vi "Z900_navX_Get_SystemInformation_Status.vi"(8 "error in (no error)":errorcluster, 11 "navX Device":T4={"Interface"={"Protocol"=enum."SERIAL", "Update Rate (4Hz-100Hz)"=4, "navX Open TypeDef"=variant}, "Notify Packet"=refnum, "Loop VI Refnum"=refnum, "Ready to Close Occurrence Refnum"=refnum} {"Interface"."Update Rate (4Hz-100Hz)" min=4 max=60 step=1}) -> (0 "error out":errorcluster, 1 "Connected":bool, 2 "Status":T3 {"OP Status" items=["INITIALIZING", "SELFTEST_IN_PROGRESS", "ERROR", "IMU_AUTOCAL_IN_PROGRESS", "NORMAL"]; "Calibration Status" items=["IMU_CAL_STATE_MASK"=3, "IMU_CAL_STATE_INPROGRESS"=0, "IMU_CAL_STATE_ACCUMULATE"=1, "IMU_CAL_STATE_COMPLETE"=2]}, 3 "navX Device":T4={"Interface"={"Protocol"=enum."SERIAL", "Update Rate (4Hz-100Hz)"=4, "navX Open TypeDef"=variant}, "Notify Packet"=refnum, "Loop VI Refnum"=refnum, "Ready to Close Occurrence Refnum"=refnum} {"Interface"."Update Rate (4Hz-100Hz)" min=4 max=60 step=1})   [LabVIEW 2015, in "Apple Pi Gyro Library.lvlib" / "navX Library v2.lvlib"]
doc: "This navX VI returns the current status of the navX."
uses:
  navX Library v2.lvlib
  TypeDefs/Z900_navX_DeviceTypeDef.ctl
  TypeDefs/Z900_navX_ProtocolTypeDef.ctl
  TypeDefs/Z900_navX_NotifyPacketTypeDef.ctl
  TypeDefs/Z900_navX_ActionTypeDef.ctl
  TypeDefs/Flags/Z900_navX_Flags_OpStatusTypeDef.ctl
  TypeDefs/Flags/Z900_navX_Flags_CalibrationStatusTypeDef.ctl
  TypeDefs/Z900_navX_DeviceRegisters.ctl
  TypeDefs/Flags/Z900_navX_Flags_SelfTestStatusTypeDef.ctl
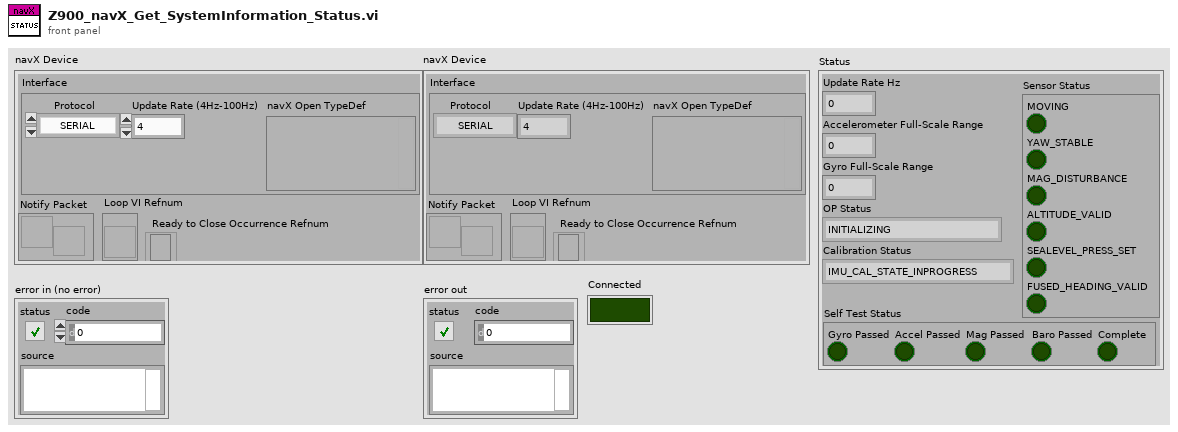
[diagram p1: front panel]
types:
  T1 = typedef "Apple Pi Gyro Library.lvlib/navX Library v2.lvlib/Z900_navX_Flags_OpStatusTypeDef.ctl" = u8
  T2 = typedef "Apple Pi Gyro Library.lvlib/navX Library v2.lvlib/Z900_navX_Flags_CalibrationStatusTypeDef.ctl" = u8
  T3 = cluster{"Update Rate Hz":u8, "Accelerometer Full-Scale Range":u8, "Gyro Full-Scale Range":u16, "OP Status":T1, "Calibration Status":T2, "Sensor Status":cluster{"MOVING":bool, "YAW_STABLE":bool, "MAG_DISTURBANCE":bool, "ALTITUDE_VALID":bool, "SEALEVEL_PRESS_SET":bool, "FUSED_HEADING_VALID":bool}, "Self Test Status":cluster{"Gyro Passed":bool, "Accel Passed":bool, "Mag Passed":bool, "Baro Passed":bool, "Complete":bool}}
  T4 = typedef "Apple Pi Gyro Library.lvlib/navX Library v2.lvlib/Z900_navX_DeviceTypeDef.ctl" = cluster{"Interface":cluster{"Protocol":T5, "Update Rate (4Hz-100Hz)":u8, "navX Open TypeDef":variant}, "Notify Packet":refnum<notifier>, "Loop VI Refnum":refnum<vi>, "Ready to Close Occurrence Refnum":refnum<k4>}
  T5 = typedef "Apple Pi Gyro Library.lvlib/navX Library v2.lvlib/Z900_navX_ProtocolTypeDef.ctl" = enum16{"SERIAL", "I2C", "SPI"}
  T6 = cluster{"MOVING":bool, "YAW_STABLE":bool, "MAG_DISTURBANCE":bool, "ALTITUDE_VALID":bool, "SEALEVEL_PRESS_SET":bool, "FUSED_HEADING_VALID":bool}
  T7 = typedef "Apple Pi Gyro Library.lvlib/navX Library v2.lvlib/Z900_navX_DeviceRegisters.ctl" = u8
  T8 = cluster{"Gyro Passed":bool, "Accel Passed":bool, "Mag Passed":bool, "Baro Passed":bool, "Complete":bool}
  T9 = typedef "Apple Pi Gyro Library.lvlib/navX Library v2.lvlib/Z900_navX_Flags_SelfTestStatusTypeDef.ctl" = u8
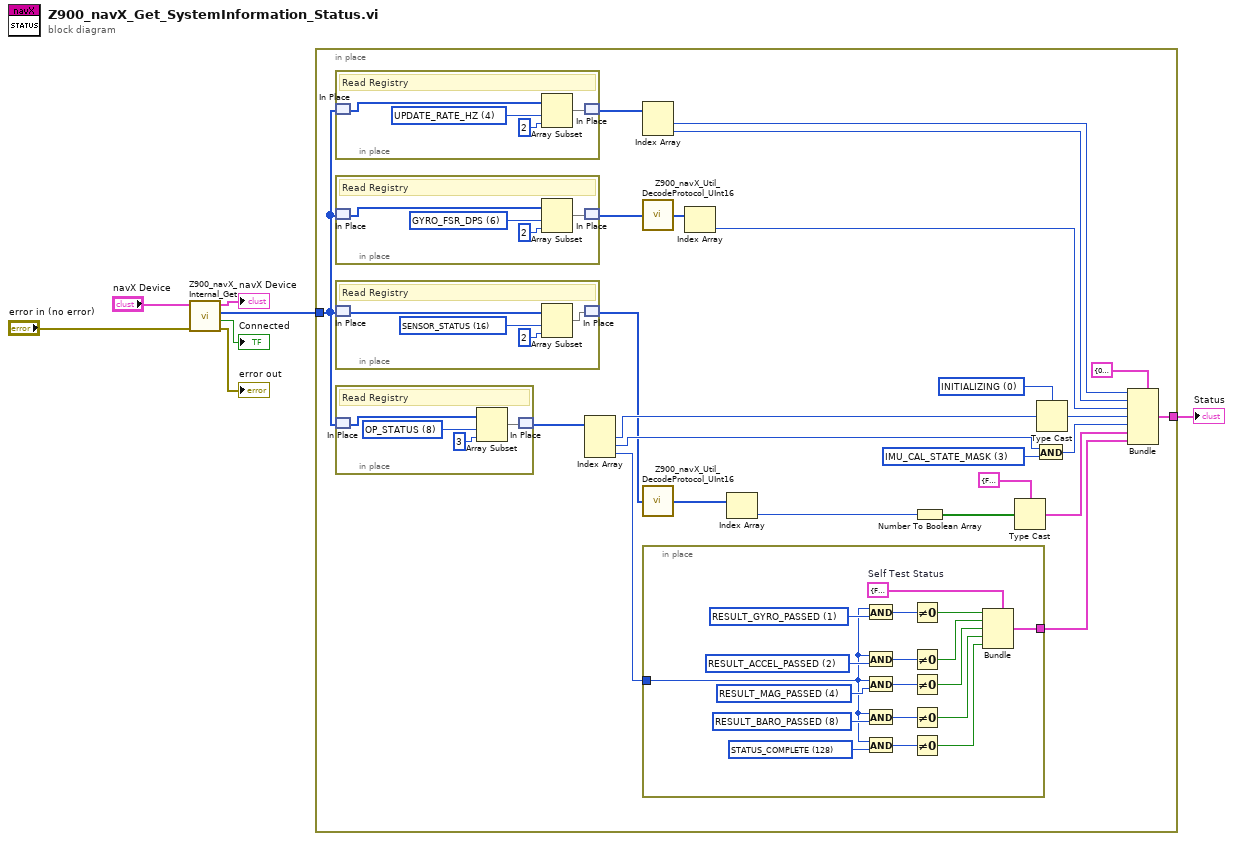
[diagram p0: block diagram]
diagram:
  n1 = call "Z900_navX_Internal_Get.vi"("error in (no error)"="error in (no error)", "navX Device"="navX Device") -> ("error out"=→"error out":errorcluster, "Connected"=→"Connected":bool, "Registry"=w3:u8[], "navX Device"=→"navX Device":T4)  [unwired: 6 in]
  n2 = in-place {
    in-place-border: w3 -> [w16]
    in-place-border: [w23] -> w1
    w27 = T2 3 items=["IMU_CAL_STATE_MASK"=3, "IMU_CAL_STATE_INPROGRESS"=0, "IMU_CAL_STATE_ACCUMULATE"=1, "IMU_CAL_STATE_COMPLETE"=2] ("CalibrationStatus")
    w29 = T1 0 items=["INITIALIZING", "SELFTEST_IN_PROGRESS", "ERROR", "IMU_AUTOCAL_IN_PROGRESS", "NORMAL"] ("OP Status")
    n3 = in-place {
      w52 = T7 4 items=["WHOAMI"=0, "HW_REV"=1, "FW_VER_MAJOR"=2, "FW_VER_MINOR"=3, "UPDATE_RATE_HZ"=4, "ACCEL_FSR_G"=5, "GYRO_FSR_DPS"=6, "OP_STATUS"=8, "CAL_STATUS"=9, "SELFTEST_STATUS"=10, "CAPABILITY_FLAGS_L"=11, "CAPABILITY_FLAGS_H"=12, "SENSOR_STATUS"=16, "TIMESTAMP"=18, "YAW"=22, "ROLL"=24, "PITCH"=26, "HEADING"=28, "FUSED_HEADING"=30, "ALTITUDE_I"=32, "ALTITUDE_D"=34, "LINERA_ACC_X"=36, "LINERA_ACC_Y"=38, "LINERA_ACC_Z"=40, "QUAT_W"=42, "QUAT_X"=44, "QUAT_Y"=46, "QUAT_Z"=48, "MPU_TEMP_C"=50, "GYRO_X"=52, "GYRO_Y"=54, "GYRO_Z"=56, "ACC_X"=58, "ACC_Y"=60, "ACC_Z"=62, "MAG_X"=64, "MAG_Y"=66, "MAG_Z"=68, "PRESSURE_I"=70, "PRESSURE_D"=72, "PRESSURE_TEMP"=74, "YAW_OFFSET"=76, "QUAT_OFFSET_W"=78, "QUAT_OFFSET_X"=80, "QUAT_OFFSET_Y"=82, "QUAT_OFFSET_Z"=84, "INTEGRATION_CONTROL"=86, "VELOCITY_X"=88, "VELOCITY_Y"=92, "VELOCITY_Z"=96, "DISPLACMENT_X"=100, "DISPLACMENT_Y"=104, "DISPLACEMENT_Z"=108] ("Device Register")
      # "Read Registry"
      n4 = in-place-match #1(w16) -> (w50:u8[])
      n5 = Array Subset(array=w50, index=w52, length=2) -> (w51:u8[])
      n6 = in-place-match #1(w51) -> (w15:u8[])
    }
    n7 = in-place {
      w64 = T7 6 items=["WHOAMI"=0, "HW_REV"=1, "FW_VER_MAJOR"=2, "FW_VER_MINOR"=3, "UPDATE_RATE_HZ"=4, "ACCEL_FSR_G"=5, "GYRO_FSR_DPS"=6, "OP_STATUS"=8, "CAL_STATUS"=9, "SELFTEST_STATUS"=10, "CAPABILITY_FLAGS_L"=11, "CAPABILITY_FLAGS_H"=12, "SENSOR_STATUS"=16, "TIMESTAMP"=18, "YAW"=22, "ROLL"=24, "PITCH"=26, "HEADING"=28, "FUSED_HEADING"=30, "ALTITUDE_I"=32, "ALTITUDE_D"=34, "LINERA_ACC_X"=36, "LINERA_ACC_Y"=38, "LINERA_ACC_Z"=40, "QUAT_W"=42, "QUAT_X"=44, "QUAT_Y"=46, "QUAT_Z"=48, "MPU_TEMP_C"=50, "GYRO_X"=52, "GYRO_Y"=54, "GYRO_Z"=56, "ACC_X"=58, "ACC_Y"=60, "ACC_Z"=62, "MAG_X"=64, "MAG_Y"=66, "MAG_Z"=68, "PRESSURE_I"=70, "PRESSURE_D"=72, "PRESSURE_TEMP"=74, "YAW_OFFSET"=76, "QUAT_OFFSET_W"=78, "QUAT_OFFSET_X"=80, "QUAT_OFFSET_Y"=82, "QUAT_OFFSET_Z"=84, "INTEGRATION_CONTROL"=86, "VELOCITY_X"=88, "VELOCITY_Y"=92, "VELOCITY_Z"=96, "DISPLACMENT_X"=100, "DISPLACMENT_Y"=104, "DISPLACEMENT_Z"=108] ("Device Register")
      # "Read Registry"
      n8 = in-place-match #2(w16) -> (w62:u8[])
      n9 = Array Subset(array=w62, index=w64, length=2) -> (w63:u8[])
      n10 = in-place-match #2(w63) -> (w17:u8[])
    }
    n11 = in-place {
      w56 = T7 16 items=["WHOAMI"=0, "HW_REV"=1, "FW_VER_MAJOR"=2, "FW_VER_MINOR"=3, "UPDATE_RATE_HZ"=4, "ACCEL_FSR_G"=5, "GYRO_FSR_DPS"=6, "OP_STATUS"=8, "CAL_STATUS"=9, "SELFTEST_STATUS"=10, "CAPABILITY_FLAGS_L"=11, "CAPABILITY_FLAGS_H"=12, "SENSOR_STATUS"=16, "TIMESTAMP"=18, "YAW"=22, "ROLL"=24, "PITCH"=26, "HEADING"=28, "FUSED_HEADING"=30, "ALTITUDE_I"=32, "ALTITUDE_D"=34, "LINERA_ACC_X"=36, "LINERA_ACC_Y"=38, "LINERA_ACC_Z"=40, "QUAT_W"=42, "QUAT_X"=44, "QUAT_Y"=46, "QUAT_Z"=48, "MPU_TEMP_C"=50, "GYRO_X"=52, "GYRO_Y"=54, "GYRO_Z"=56, "ACC_X"=58, "ACC_Y"=60, "ACC_Z"=62, "MAG_X"=64, "MAG_Y"=66, "MAG_Z"=68, "PRESSURE_I"=70, "PRESSURE_D"=72, "PRESSURE_TEMP"=74, "YAW_OFFSET"=76, "QUAT_OFFSET_W"=78, "QUAT_OFFSET_X"=80, "QUAT_OFFSET_Y"=82, "QUAT_OFFSET_Z"=84, "INTEGRATION_CONTROL"=86, "VELOCITY_X"=88, "VELOCITY_Y"=92, "VELOCITY_Z"=96, "DISPLACMENT_X"=100, "DISPLACMENT_Y"=104, "DISPLACEMENT_Z"=108] ("Device Register")
      # "Read Registry"
      n12 = in-place-match #3(w16) -> (w54:u8[])
      n13 = Array Subset(array=w54, index=w56, length=2) -> (w55:u8[])
      n14 = in-place-match #3(w55) -> (w22:u8[])
    }
    n15 = in-place {
      w60 = T7 8 items=["WHOAMI"=0, "HW_REV"=1, "FW_VER_MAJOR"=2, "FW_VER_MINOR"=3, "UPDATE_RATE_HZ"=4, "ACCEL_FSR_G"=5, "GYRO_FSR_DPS"=6, "OP_STATUS"=8, "CAL_STATUS"=9, "SELFTEST_STATUS"=10, "CAPABILITY_FLAGS_L"=11, "CAPABILITY_FLAGS_H"=12, "SENSOR_STATUS"=16, "TIMESTAMP"=18, "YAW"=22, "ROLL"=24, "PITCH"=26, "HEADING"=28, "FUSED_HEADING"=30, "ALTITUDE_I"=32, "ALTITUDE_D"=34, "LINERA_ACC_X"=36, "LINERA_ACC_Y"=38, "LINERA_ACC_Z"=40, "QUAT_W"=42, "QUAT_X"=44, "QUAT_Y"=46, "QUAT_Z"=48, "MPU_TEMP_C"=50, "GYRO_X"=52, "GYRO_Y"=54, "GYRO_Z"=56, "ACC_X"=58, "ACC_Y"=60, "ACC_Z"=62, "MAG_X"=64, "MAG_Y"=66, "MAG_Z"=68, "PRESSURE_I"=70, "PRESSURE_D"=72, "PRESSURE_TEMP"=74, "YAW_OFFSET"=76, "QUAT_OFFSET_W"=78, "QUAT_OFFSET_X"=80, "QUAT_OFFSET_Y"=82, "QUAT_OFFSET_Z"=84, "INTEGRATION_CONTROL"=86, "VELOCITY_X"=88, "VELOCITY_Y"=92, "VELOCITY_Z"=96, "DISPLACMENT_X"=100, "DISPLACMENT_Y"=104, "DISPLACEMENT_Z"=108] ("Device Register")
      # "Read Registry"
      n16 = in-place-match #4(w16) -> (w58:u8[])
      n17 = Array Subset(array=w58, index=w60, length=3) -> (w59:u8[])
      n18 = in-place-match #4(w59) -> (w31:u8[])
    }
    n19 = Index Array(array=w31) -> (element #1=w30:u8, element #2=w28:u8, element #3=w10:u8)  [unwired: 3 in]
    n20 = Index Array(array=w15) -> (element #1=w11:u8, element #2=w12:u8)  [unwired: 2 in]
    n21 = call "Z900_navX_Util_DecodeProtocol_UInt16.vi"("Little Endian"=w17) -> ("UInt16"=w14:u16[])
    n22 = call "Z900_navX_Util_DecodeProtocol_UInt16.vi"("Little Endian"=w22) -> ("UInt16"=w21:u16[])
    n23 = in-place {
      in-place-border: w10 -> [w39]
      in-place-border: [w32] -> w8
      w38 = T8 {"Gyro Passed"=FALSE, "Accel Passed"=FALSE, "Mag Passed"=FALSE, "Baro Passed"=FALSE, "Complete"=FALSE}  # Self Test Status
      w41 = T9 128 items=["STATUS_COMPLETE"=128, "RESULT_GYRO_PASSED"=1, "RESULT_ACCEL_PASSED"=2, "RESULT_MAG_PASSED"=4, "RESULT_BARO_PASSED"=8] ("Self Test Status")
      w42 = T9 8 items=["STATUS_COMPLETE"=128, "RESULT_GYRO_PASSED"=1, "RESULT_ACCEL_PASSED"=2, "RESULT_MAG_PASSED"=4, "RESULT_BARO_PASSED"=8] ("Self Test Status")
      w45 = T9 4 items=["STATUS_COMPLETE"=128, "RESULT_GYRO_PASSED"=1, "RESULT_ACCEL_PASSED"=2, "RESULT_MAG_PASSED"=4, "RESULT_BARO_PASSED"=8] ("Self Test Status")
      w46 = T9 2 items=["STATUS_COMPLETE"=128, "RESULT_GYRO_PASSED"=1, "RESULT_ACCEL_PASSED"=2, "RESULT_MAG_PASSED"=4, "RESULT_BARO_PASSED"=8] ("Self Test Status")
      w49 = T9 1 items=["STATUS_COMPLETE"=128, "RESULT_GYRO_PASSED"=1, "RESULT_ACCEL_PASSED"=2, "RESULT_MAG_PASSED"=4, "RESULT_BARO_PASSED"=8] ("Self Test Status")
      n24 = And(x=w39, y=w49) -> (x .and. y?=w48:T9)
      n25 = And(x=w39, y=w46) -> (x .and. y?=w47:T9)
      n26 = And(x=w39, y=w45) -> (x .and. y?=w44:T9)
      n27 = And(x=w39, y=w42) -> (x .and. y?=w43:T9)
      n28 = And(x=w39, y=w41) -> (x .and. y?=w40:T9)
      n29 = Not Equal To 0?(x=w48) -> (x != 0?=w37:bool)
      n30 = Not Equal To 0?(x=w47) -> (x != 0?=w36:bool)
      n31 = Not Equal To 0?(x=w44) -> (x != 0?=w35:bool)
      n32 = Not Equal To 0?(x=w43) -> (x != 0?=w34:bool)
      n33 = Not Equal To 0?(x=w40) -> (x != 0?=w33:bool)
      n34 = Bundle(cluster=w38, "Gyro Passed"=w37, "Accel Passed"=w36, "Mag Passed"=w35, "Baro Passed"=w34, "Complete"=w33) -> (w32:T8)
    }
    n35 = Index Array(array=w14) -> (element=w13:u16)  [unwired: 1 in]
    n36 = Index Array(array=w21) -> (element=w20:u16)  [unwired: 1 in]
    n37 = Number To Boolean Array(number=w20) -> (Boolean array=w19:bool[])
    n38 = Type Cast(type=T6 {"MOVING"=FALSE, "YAW_STABLE"=FALSE, "MAG_DISTURBANCE"=FALSE, "ALTITUDE_VALID"=FALSE, "SEALEVEL_PRESS_SET"=FALSE, "FUSED_HEADING_VALID"=FALSE} ("NAVX_SENSOR_STATUS"), x=w19) -> (*(type *) &x=w9:T6)
    n39 = And(x=w28, y=w27) -> (x .and. y?=w24:T2)
    n40 = Type Cast(type=w29, x=w30) -> (*(type *) &x=w25:T1)
    n41 = Bundle(cluster=T3 {"Update Rate Hz"=0, "Accelerometer Full-Scale Range"=0, "Gyro Full-Scale Range"=0, "OP Status"=0, "Calibration Status"=3, "Sensor Status"={"MOVING"=FALSE, "YAW_STABLE"=FALSE, "MAG_DISTURBANCE"=FALSE, "ALTITUDE_VALID"=FALSE, "SEALEVEL_PRESS_SET"=FALSE, "FUSED_HEADING_VALID"=FALSE}, "Self Test Status"={"Gyro Passed"=FALSE, "Accel Passed"=FALSE, "Mag Passed"=FALSE, "Baro Passed"=FALSE, "Complete"=FALSE}}, "Update Rate Hz"=w11, "Accelerometer Full-Scale Range"=w12, "Gyro Full-Scale Range"=w13, "OP Status"=w25, "Calibration Status"=w24, "Sensor Status"=w9, "Self Test Status"=w8) -> (w23:T3)
  }
  "Status" <- w1
